vi "Timer.vi"(8 "error in (no error)":errorcluster, 9 "Reset":bool, 10 "Target Time":dbl) -> (0 "error out":errorcluster, 1 "Elapsed?":bool, 2 "Elapsed Time(s)":dbl)   [LabVIEW 2018]
doc: "This VI is used as a subVI in the application Sprinkler Controller to set the servicing time of various Zones."
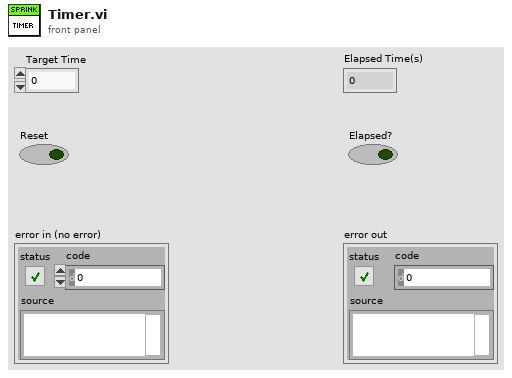
[diagram p1: front panel]
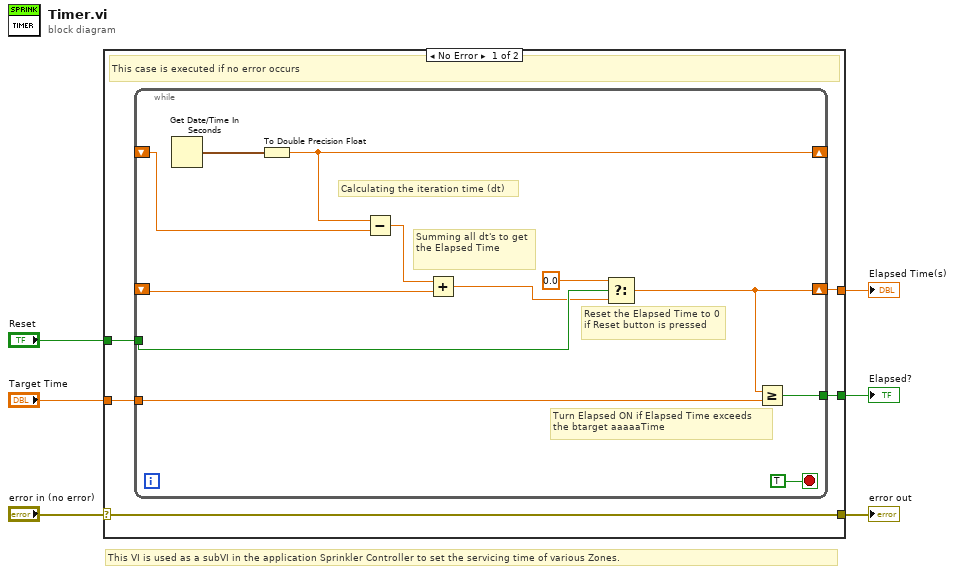
[diagram p0: block diagram]
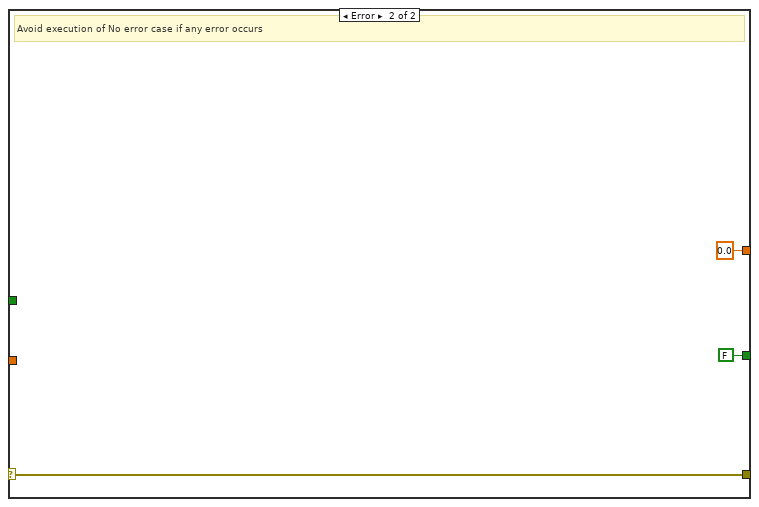
[diagram p2: hidden frame]
diagram:
  # "This VI is used as a subVI in the application Sprinkler Controller to set the servicing time of various Zones."
  n1 = case shown="No Error" "error in (no error)" {
    selector: "error in (no error)" -> [w11 w26]
    tunnel: [w11 w26] -> w2
    tunnel: "Reset" -> [w10 _]
    tunnel: "Target Time" -> [w9 _]
    tunnel: [w8 FALSE] -> w5
    tunnel: [w7 0.0 ("t")] -> w6
    frame No Error {
      # "This case is executed if no error occurs"
      n2 = while {
        shift-right: [w21] -> _
        shift-left: _ -> [w20]
        shift-right: [w14] -> w7
        shift-left: _ -> [w18]
        tunnel: w10 -> [w17]
        tunnel: w9 -> [w13]
        tunnel: [w12] -> w8
        stop <- TRUE stop-if-true
        # "Turn Elapsed ON if Elapsed Time exceeds \nthe btarget aaaaaTime"
        # "Reset the Elapsed Time to 0 if Reset button is pressed"
        # "Summing all dt's to get the Elapsed Time"
        # "Calculating the iteration time (dt)"
        n3 = Get Date/Time In Seconds() -> (seconds since 1Jan1904=w23:timestamp)
        n4 = To Double Precision Float(number=w23) -> (double precision float=w21:dbl)
        n5 = Subtract(x=w21, y=w20) -> (x-y=w19:dbl)
        n6 = Add(x=w19, y=w18) -> (x+y=w15:dbl)
        n7 = Select(t=0.0, s=w17, f=w15) -> (s? t:f=w14:dbl)
        n8 = Greater Or Equal?(x=w14, y=w13) -> (x >= y?=w12:bool)
      }
    }
    frame Error {
      # "Avoid execution of No error case if any error occurs"
    }
  }
  "Elapsed Time(s)" <- w6
  "Elapsed?" <- w5
  "error out" <- w2
